vi "Emballage_BDD_GVF_ref.vi"(8 "Error in":errorcluster caption="Error in (no error)", 9 "Refnum Numsem":refnum<vi>, 11 "Énum":enum16{"set", "get"}(ring)=enum."get") -> (0 "Error out":errorcluster, 1 "Refnum NumSem OUT":refnum<vi>)   [LabVIEW 2020]
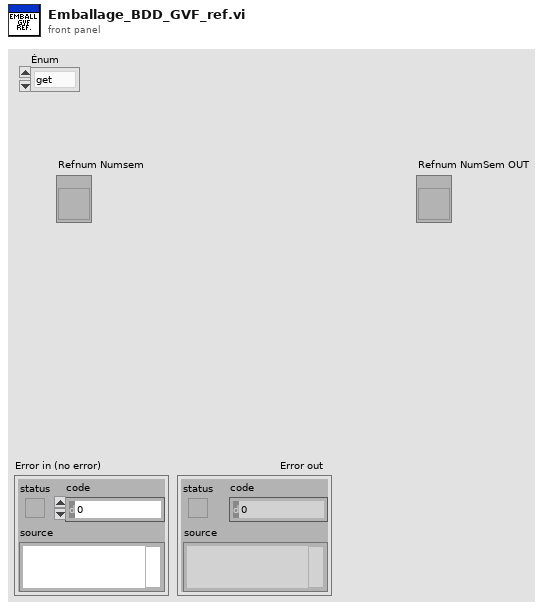
[diagram p1: front panel]
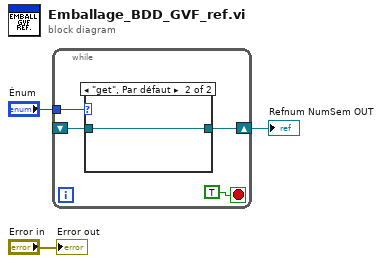
[diagram p0: block diagram]
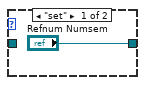
[diagram p2: hidden frame]
diagram:
  n1 = while {
    tunnel: "Énum" -> [w6]
    shift-right: [w5] -> w1
    shift-left: _ -> [w4]
    stop <- TRUE stop-if-true
    n2 = case shown="\"get\", Par défaut" w6 {
      tunnel: ["Refnum Numsem" w9] -> w5
      tunnel: w4 -> [_ w9]
      frame "set" {
      }
      frame "get", Default {
      }
    }
  }
  "Refnum NumSem OUT" <- w1
  "Error out" <- "Error in"
